vi "Team Name.vi"(8 "error in (no error)":errorcluster, 11 "MyTeam in":refnum<class "MyTeam.lvclass">) -> (0 "error out":errorcluster, 3 "MyTeam out":refnum<class "MyTeam.lvclass">, 7 "Team Name":string)   [LabVIEW 2020, in "SquareTeam.lvlib" / "MyTeam.lvclass"]
uses:
  MyTeam.lvclass
  MyTeam.lvclass/MyTeam.ctl
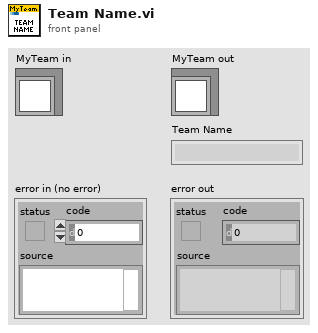
[diagram p1: front panel]
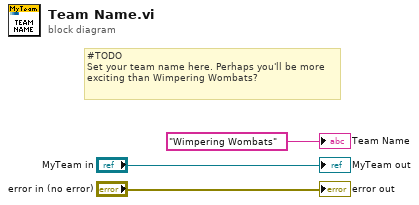
[diagram p0: block diagram]
diagram:
  # "#TODO\nSet your team name here. Perhaps you'll be more exciting than Wimpering Wombats?"
  "error out" <- "error in (no error)"
  "MyTeam out" <- "MyTeam in"
  "Team Name" <- "Wimpering Wombats" ("Team Name")
